vi "writeLogFileHeader.vi"(8 "error out 2":errorcluster, 11 "Protocol_Generic out":refnum<class "Protocol_Logging.lvclass">) -> (0 "error out":errorcluster, 3 "Protocol_Generic out 2":refnum<class "Protocol_Logging.lvclass">)   [LabVIEW 2011, in "Protocol_Logging.lvclass"]
uses:
  Protocol_Logging.lvclass
  Protocol_Logging.lvclass/Protocol_Logging.ctl
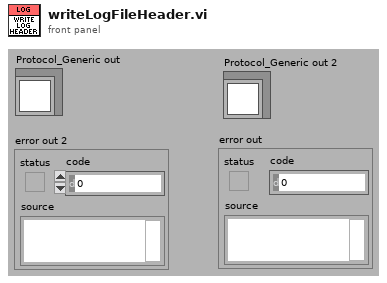
[diagram p1: front panel]
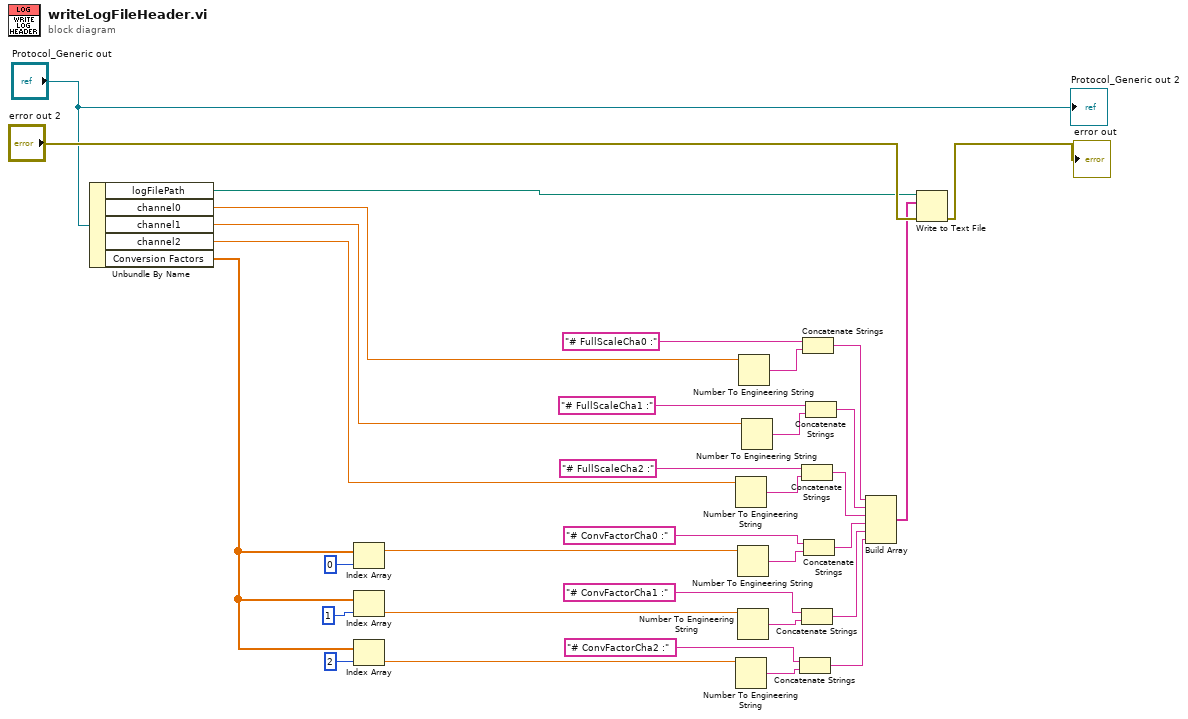
[diagram p0: block diagram]
diagram:
  n1 = Unbundle By Name("Protocol_Generic out") -> ("logFilePath"=w1:path, "channel0"=w22:dbl, "channel1"=w23:dbl, "channel2"=w24:dbl, "Conversion Factors"=w28:dbl[])
  n2 = Index Array(array=w28, index=0) -> (element=w29:dbl)
  n3 = Index Array(array=w28, index=1) -> (element=w30:dbl)
  n4 = Index Array(array=w28, index=2) -> (element=w31:dbl)
  n5 = Number To Engineering String(4:w24) -> (0:w12:string)  [unwired: 3 in]
  n6 = Number To Engineering String(4:w31) -> (0:w20:string)  [unwired: 3 in]
  n7 = Number To Engineering String(4:w29) -> (0:w14:string)  [unwired: 3 in]
  n8 = Number To Engineering String(4:w30) -> (0:w17:string)  [unwired: 3 in]
  n9 = Number To Engineering String(4:w22) -> (0:w6:string)  [unwired: 3 in]
  n10 = Number To Engineering String(4:w23) -> (0:w8:string)  [unwired: 3 in]
  n11 = Concatenate Strings("# ConvFactorCha2 :", w20) -> (w21:string)
  n12 = Concatenate Strings("# FullScaleCha2 :", w12) -> (w11:string)
  n13 = Concatenate Strings("# ConvFactorCha1 :", w17) -> (w18:string)
  n14 = Concatenate Strings("# FullScaleCha0 :", w6) -> (w4:string)
  n15 = Concatenate Strings("# ConvFactorCha0 :", w14) -> (w15:string)
  n16 = Concatenate Strings("# FullScaleCha1 :", w8) -> (w9:string)
  n17 = Build Array(w4, w9, w11, w15, w18, w21) -> (w3:string[])
  n18 = Write to Text File(file (use dialog)=w1, text=w3, error in="error out 2") -> (error out=→"error out":errorcluster)  [unwired: 1 in, 2 out]
  "Protocol_Generic out 2" <- "Protocol_Generic out"
